vi "Joystick Global 6740.vi"() -> ()   [LabVIEW 2016]
panel:
  in  "Right X3D POVs":i16[](array[numeric])
  out "Right 12":bool
  out "Right 11":bool
  out "Right 10":bool
  out "Right 9":bool
  out "Right 8":bool
  out "Right 7":bool
  out "Right 6":bool
  out "Right 5":bool
  out "Right 4":bool
  out "Right 3":bool
  out "Right 2":bool
  out "Right 1":bool
  in  "Right Joystick Slider":dbl
  in  "Right Joystick Y Axis":dbl
  in  "Right Joystick Z Axis":dbl
  in  "Right Joystick X Axis":dbl
  in  "Right X3D Joystick Axis":T1
  out "Right X3D Joystick Buttons":T2
  in  "Xbox POVs":i16[](array[numeric])
  in  "Left X3D POVs":i16[](array[numeric])
  out "Left 12":bool
  out "Left 11":bool
  out "Left 10":bool
  out "Left 9":bool
  out "Left 8":bool
  out "Left 7":bool
  out "Left 6":bool
  out "Left 5":bool
  out "Left 4":bool
  out "Left 3":bool
  out "Left 2":bool
  out "Left 1":bool
  in  "Left Joystick Slider":dbl
  in  "Left Joystick Y Axis":dbl
  in  "Left Joystick Z Axis":dbl
  in  "Left Joystick X Axis":dbl
  in  "Left X3D Joystick Axis":T1
  out "Left X3D Joystick Buttons":T2
  out ".Right Joystick Button":bool
  out ".Y":bool
  out ".B":bool
  out ".Start":bool
  out ".RB":bool
  out ".Left Joystick Button":bool
  out ".Back":bool
  out ".LB":bool
  out ".X":bool
  out ".A":bool
  in  "Xbox Axis":T3
  out "Xbox Buttons":T4
  in  "Xbox Right Y":dbl
  in  "Xbox Right X":dbl
  in  "Xbox Right Trigger":dbl
  in  "Xbox Left Trigger":dbl
  in  "Xbox Left Y":dbl
  in  "Xbox Left X":dbl
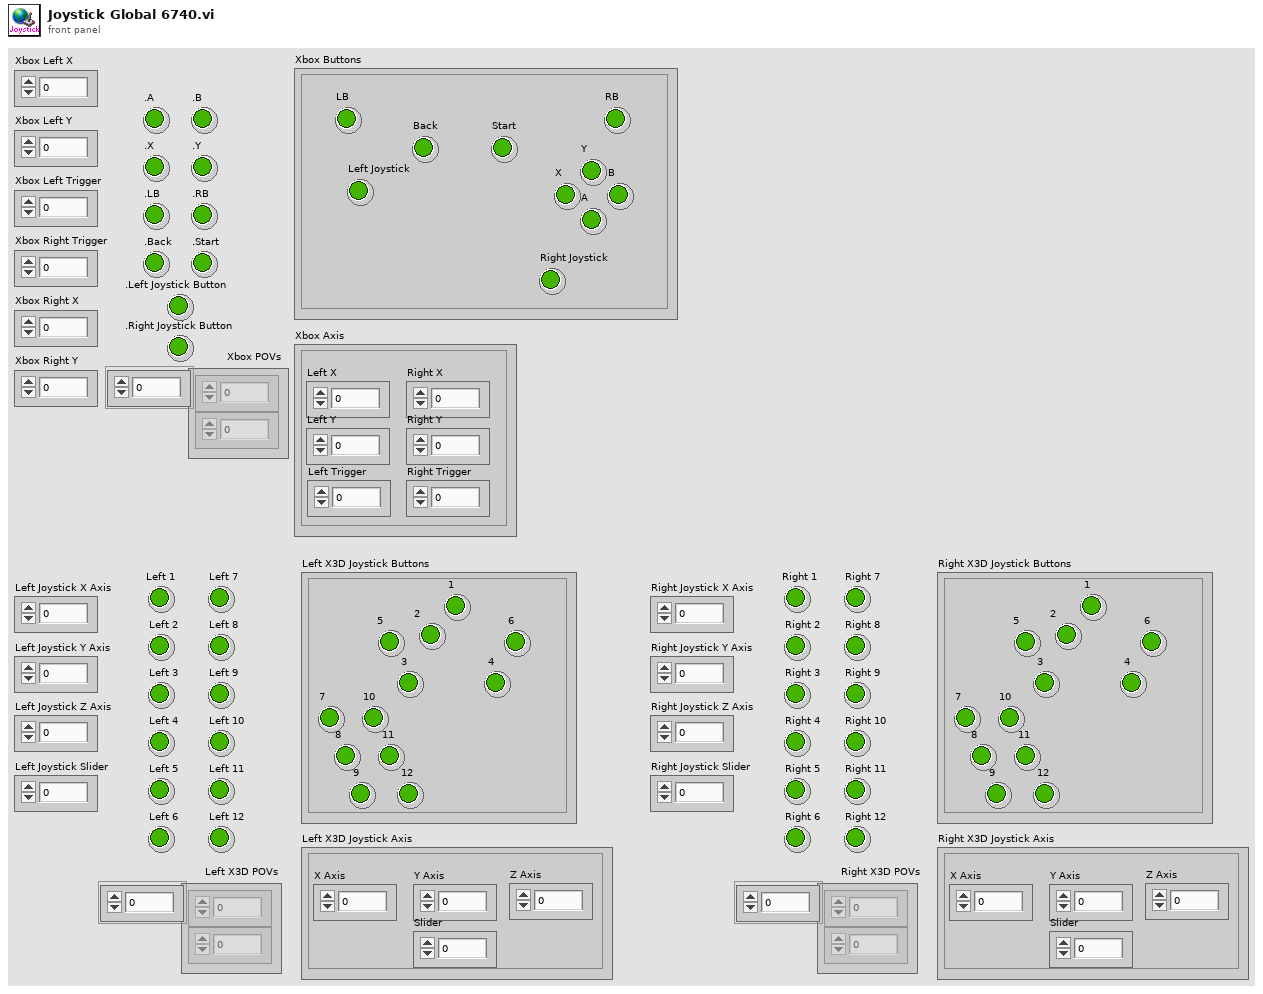
[diagram p1: front panel]
types:
  T1 = cluster{"X Axis":dbl, "Y Axis":dbl, "Z Axis":dbl, "Slider":dbl}
  T2 = cluster{" 1":bool, " 2":bool, " 3":bool, " 5":bool, " 4":bool, " 6":bool, "7":bool, "8":bool, " 9":bool, "10":bool, " 11":bool, " 12":bool}
  T3 = cluster{"Left X":dbl, "Left Y":dbl, "Left Trigger":dbl, "Right Trigger":dbl, "Right X":dbl, "Right Y":dbl}
  T4 = cluster{"A":bool, "B":bool, "X":bool, "Y":bool, "LB":bool, "RB":bool, "Back":bool, "Start":bool, "Left Joystick":bool, "Right Joystick":bool}
diagram:
